vi "DB Search CMD.vi"(8 "error in (no error)":errorcluster, 9 "SQL CMD":string, 10 "Actor Name":string, 11 "DB_Search in":refnum<class "DB_Search.lvclass">) -> (0 "error out":errorcluster, 3 "DB_Search out":refnum<class "DB_Search.lvclass">)   [LabVIEW 2021, in "DB_SearchCMD.lvlib" / "DB_Search.lvclass"]
uses:
  <userlib>/John_Lib/Interfaces/DB_Search/DB_Search.lvclass
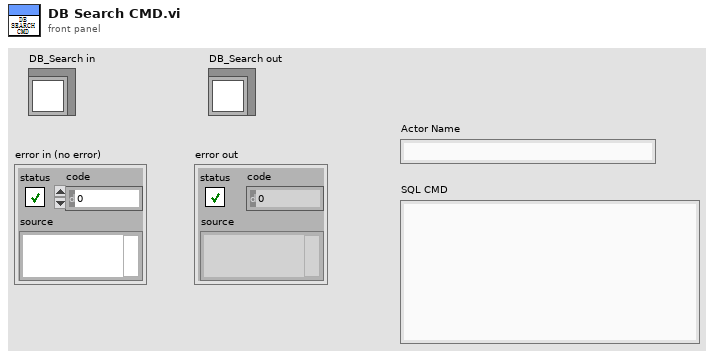
[diagram p1: front panel]
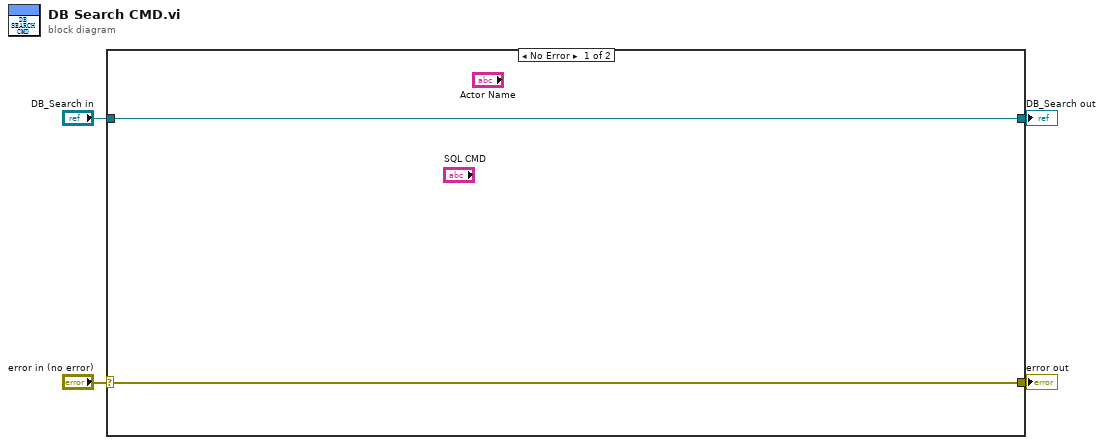
[diagram p0: block diagram]
diagram:
  n1 = case shown="No Error" "error in (no error)" {
    selector: "error in (no error)" -> [w5 w8]
    tunnel: [w5 w8] -> w3
    tunnel: [w6 w7] -> w1
    tunnel: "DB_Search in" -> [w6 w7]
    frame No Error {
    }
    frame Error {
    }
  }
  "error out" <- w3
  "DB_Search out" <- w1
